vi "getChannelType.vi"(8 "error in (no error)":errorcluster, 11 "StaticOutputEditor in":refnum<class "StaticOutputEditor.lvclass">) -> (0 "error out":errorcluster, 2 "channel_type":enum16{"ao", "do", "ai", "di", "rf"}(ring), 3 "StaticOutputEditor out":refnum<class "StaticOutputEditor.lvclass">)   [LabVIEW 2011, in "Views.lvlib" / "ScriptEditor.lvlib" / "StaticOutputEditor.lvclass"]
uses:
  StaticOutputEditor.lvclass
  StaticOutputEditor.lvclass/StaticOutputEditor.ctl
  Tools/DatabaseHelpers/Database Objects/ChannelArray/ChannelArray.lvclass
  Tools/DatabaseHelpers/Database Objects/Channel/Channel.lvclass
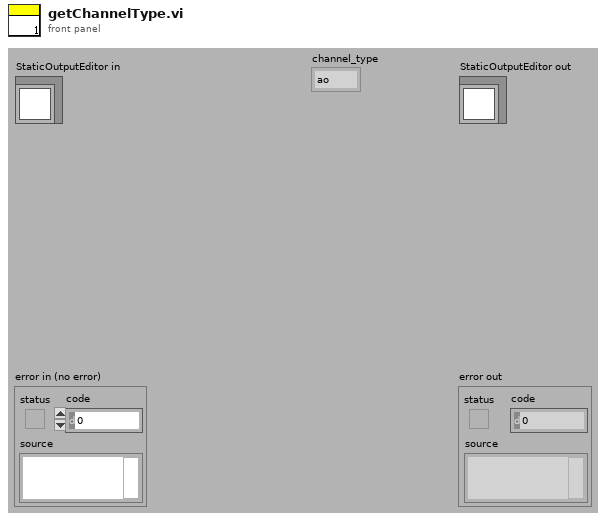
[diagram p1: front panel]
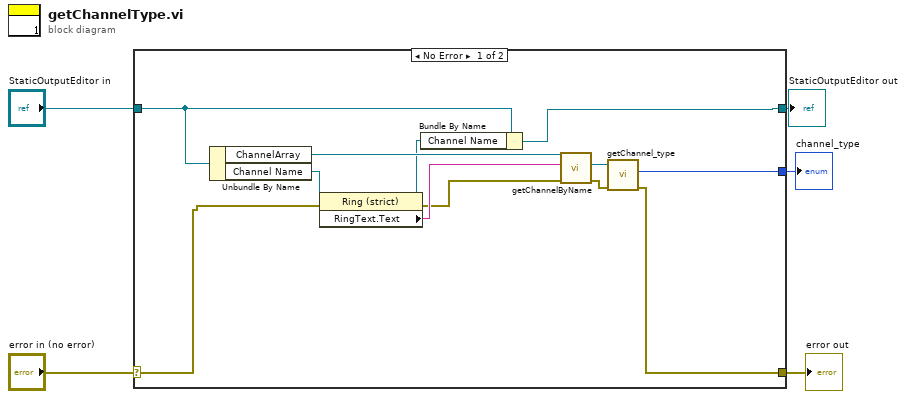
[diagram p0: block diagram]
diagram:
  n1 = case shown="No Error" "error in (no error)" {
    selector: "error in (no error)" -> [w8 w19]
    tunnel: [w7 w19] -> w4
    tunnel: [w10 w18] -> w2
    tunnel: "StaticOutputEditor in" -> [w6 w18]
    tunnel: [w9 _] -> w1
    frame No Error {
      n2 = Unbundle By Name(w6) -> ("ChannelArray"=w16:refnum<class "ChannelArray.lvclass">, "Channel Name"=w17:refnum<vi>)
      n3 = property class="Ring (strict)"(reference=w17, error in=w8) -> (reference out=w11:refnum<vi>, error out=w14:errorcluster, "RingText.Text"=w15:string)
      n4 = Bundle By Name(cluster=w6, "Channel Name"=w11) -> (w10:refnum<class "StaticOutputEditor.lvclass">)
      n5 = call-dynamic "getChannelByName.vi"("error in (no error)"=w14, "channel_name"=w15, "ChannelArray in"=w16) -> ("error out"=w12:errorcluster, "Channel"=w13:refnum<class "Channel.lvclass">)  [unwired: 5 in, 2 out]
      n6 = call "getChannel_type.vi"("error in (no error)"=w12, "Channel.lvclass in"=w13) -> ("error out"=w7:errorcluster, "channel_type"=w9:enum16{"ao", "do", "ai", "di", "rf"})  [unwired: 7 in, 1 out]
    }
    frame Error {
    }
  }
  "error out" <- w4
  "StaticOutputEditor out" <- w2
  "channel_type" <- w1
